vi "Self-Test.vi"(8 "error in (no error)":errorcluster, 11 "VISA resource name":refnum<visa-resource-name>) -> (0 "error out":errorcluster {"code" format="%.0x"}, 1 "Self-Test Result Message":string, 2 "Self-Test Result Code":i32, 3 "VISA resource name out":refnum<visa-resource-name>)   [LabVIEW 2014, in "Agilent PSG MXG Series.lvlib"]
doc: "Runs the instrument's self-test routine and returns the test results."
uses:
  Agilent PSG MXG Series.lvlib
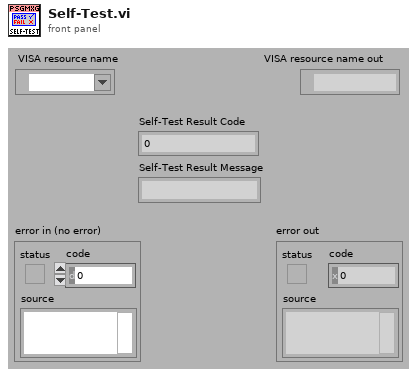
[diagram p1: front panel]
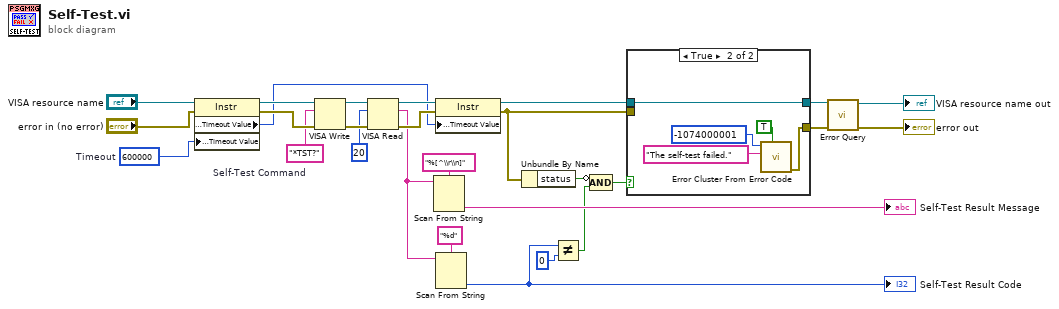
[diagram p0: block diagram]
diagram:
  w18 = u32 600000  # Timeout
  w14 = "*TST?"  # Self-Test Command
  n1 = property class="Instr"(reference="VISA resource name", error in="error in (no error)", "General Settings:Timeout Value"=w18) -> (reference out=w16:refnum<visa-resource-name>, error out=w17:errorcluster, "General Settings:Timeout Value"=w15:u32)
  n2 = VISA Write(VISA resource name=w16, write buffer=w14, error in (no error)=w17) -> (VISA resource name out=w23:refnum<visa-resource-name>, error out=w22:errorcluster)  [unwired: 1 out]
  n3 = VISA Read(VISA resource name=w23, byte count=u32 20 ("byte count (20)"), error in (no error)=w22) -> (VISA resource name out=w25:refnum<visa-resource-name>, read buffer=w20:string, error out=w24:errorcluster)  [unwired: 1 out]
  n4 = Scan From String(format string="%[^\\r\\n]" ("Format String"), input string=w20) -> (output 1=→"Self-Test Result Message":string)  [unwired: 2 in, 4 out]
  n5 = property class="Instr"(reference=w25, error in=w24, "General Settings:Timeout Value"=w15) -> (reference out=w13:refnum<visa-resource-name>, error out=w12:errorcluster)
  n6 = Scan From String(format string="%d", input string=w20) -> (output 1=w6:i32)  [unwired: 2 in, 4 out]
  "Self-Test Result Code" <- w6
  n7 = Unbundle By Name(w12) -> ("status"=w8:bool)
  n8 = Not Equal?(x=w6, y=0) -> (x != y?=w9:bool)
  n9 = Compound Arithmetic op=AND(invert w8, w9) -> (w7:bool)
  n10 = case shown="True" w7 {
    tunnel: w13 -> [w29 w34]
    tunnel: w12 -> [w28 _]
    tunnel: [w28 w30] -> w11
    tunnel: [w29 w34] -> w10
    frame False {
    }
    frame True {
      n11 = call "Error Cluster From Error Code.vi"("show call chain? (False)"=TRUE, "error message (\"\")"="The self-test failed." ("Source (VI Name)"), "error code (0)"=-1074000001 ("Code")) -> ("error out"=w30:errorcluster)  [unwired: 1 in, 5 out]
    }
  }
  n12 = call "Error Query.vi"("error in (no error)"=w11, "VISA resource name"=w10) -> ("error out"=→"error out":errorcluster, "VISA resource name out"=→"VISA resource name out":refnum<visa-resource-name>)  [unwired: 8 out]
